vi "Configure External Trigger.vi"(8 "error in (no error)":errorcluster, 10 "External Trigger Function (Rise)":u16(ring) items=["Rise", "Fall"], 11 "VISA resource name":refnum<visa-resource-name>) -> (0 "error out":errorcluster, 3 "VISA resource name out":refnum<visa-resource-name>)   [LabVIEW 2020, in "Library Instrument & Equipement.lvlib" / "Library Multimeter.lvlib" / "RIGOL DM3058.lvlib"]
doc: "Configures the External Trigger Function."
uses:
  RIGOL DM3058.lvlib
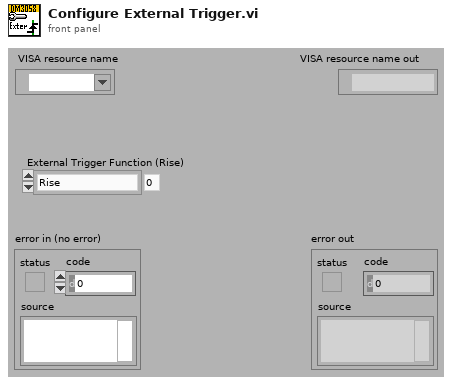
[diagram p1: front panel]
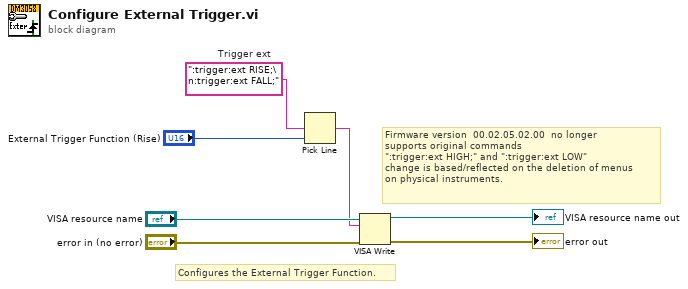
[diagram p0: block diagram]
diagram:
  w6 = ":trigger:ext RISE;\n:trigger:ext FALL;"  # Trigger ext
  # "Firmware version  00.02.05.02.00  no longer\nsupports original commands\n\":trigger:ext HIGH;\" and \":trigger:ext LOW\" \nchange is based/reflected on the deletion of menus \non physical instruments."
  # "Configures the External Trigger Function."
  n1 = Pick Line(multi-line string=w6, line index="External Trigger Function (Rise)") -> (output string=w3:string)  [unwired: 1 out]
  n2 = VISA Write(VISA resource name="VISA resource name", write buffer=w3, error in (no error)="error in (no error)") -> (VISA resource name out=→"VISA resource name out":refnum<visa-resource-name>, error out=→"error out":errorcluster)  [unwired: 1 out]
